vi "Get Profile Element Cnt.vi"(4 "Profile Info":T1={"Profile Cnt"=1, "Envelope"=FALSE, " Profile Data Point"=0, " X Start"=0, " X Pitch"=0}) -> (1 "Element Cnt[4]":u16[](array[numeric]))   [LabVIEW 2014, in "Keyence LJ-V7000.lvlib"]
uses:
  Keyence LJ-V7000.lvlib
  Public/Clusters/Profile Info.ctl
panel:
  # "Head A Max"
  # "Head B Max"
  # "Head A min"
  # "Head B Min"
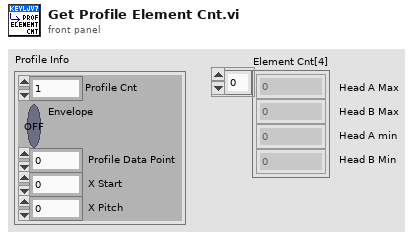
[diagram p1: front panel]
types:
  T1 = typedef "Keyence LJ-V7000.lvlib/Profile Info.ctl" = cluster{"Profile Cnt":u8, "Envelope":bool, " Profile Data Point":u16, " X Start":i32, " X Pitch":i32}
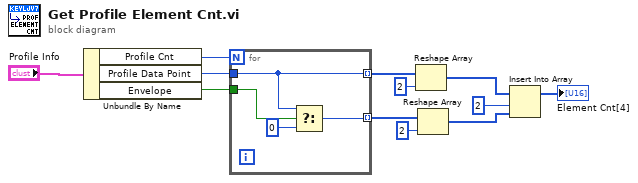
[diagram p0: block diagram]
diagram:
  n1 = Unbundle By Name("Profile Info") -> ("Profile Cnt"=w11:u8, "Profile Data Point"=w10:u16, "Envelope"=w9:bool)
  n2 = for {
    N: w11 -> [_]
    tunnel: w10 -> [w14]
    tunnel: [w14] -> w4 mode=indexing
    tunnel: w9 -> [w16]
    tunnel: [w13] -> w3 mode=indexing
    n3 = Select(t=w14, s=w16, f=u32 0) -> (s? t:f=w13:u32)
  }
  n4 = Reshape Array(w4, 2 ("次元サイズ")) -> (w6:u16[])
  n5 = Reshape Array(w3, 2 ("次元サイズ")) -> (w2:u32[])
  n6 = Insert Into Array(array=w6, index=2 ("指標"), new element=w2) -> (→"Element Cnt[4]":u16[])
